vi "rocket fuel system start.vi"() -> ()   [LabVIEW 2017]
uses:
  typedefs/fuel tank.ctl
  typedefs/horiz oxidizer valve.ctl
  typedefs/oxidizer tank.ctl
  typedefs/vertical fuel valve.ctl
  typedefs/vertical oxidizer valve.ctl
  typedefs/horiz fuel valve.ctl
  typedefs/user controls.ctl
  typedefs/system state.ctl
  typedefs/sysyem status.ctl
  typedefs/rocket system warnings.ctl
panel:
  out "fuel leak w":bool
  out "fuel over w":bool
  out "system status":T1=enum."Empty & Closed"
  out "lox leak w":bool
  out "LOX over w":bool
  in  "rocket controls":T2
  out "ignition":bool
  in  "fuel leak":bool
  in  "LOX leak":bool caption="oxidizer leak"
  in  "fuel over":bool
  in  "LOX over":bool caption="oxidizer overpress"
  out "fuel dump":T3
  out "fuel return":T3
  out "fuel load":T3
  out "LOX dump":T4
  out "LOX return":T4
  out "LOX comb":T5
  out "fuel comb":T6
  out "oxidizer tank":T7 scale=0.0..100.0
  out "LOX load":T4
  out "fuel tank":T8 scale=0.0..100.0
  # "LOX\nfeed"
  # "LOX\nreturn"
  # "fuel\nfeed"
  # "fuel\nreturn"
  # "Rocket\nEngine\nFueling\nSystem\nState\nMachine"
  # "fuel\ndump"
  # "LOX\ndump"
  # "combustion\nchamber"
  # "Standard\nProcedures"
  # "Alternate\nProcedures"
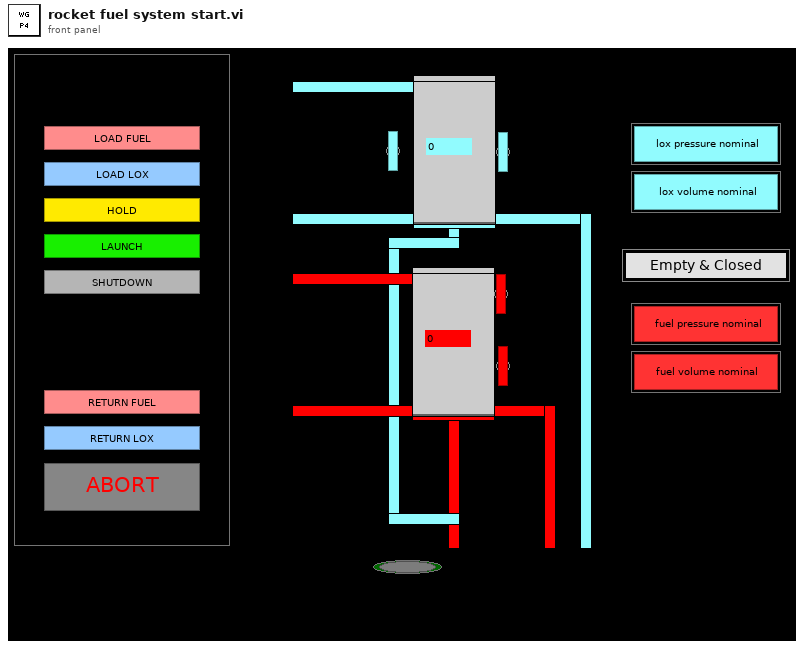
[diagram p1: front panel]
types:
  T1 = typedef "system state.ctl" = enum16{"Hold", "Empty & Closed", "Launch", "Return Fuel", "Return LOX", "Loading Lox", "Loading Fuel", "Shutdown", "Abort"}
  T2 = typedef "user controls.ctl" = cluster{"load fuel":bool, "load lox":bool, "hold":bool, "launch":bool, "shutdown":bool, "return fuel":bool, "return lox":bool, "abort":bool}
  T3 = typedef "horiz fuel valve.ctl" = u16
  T4 = typedef "horiz oxidizer valve.ctl" = u16
  T5 = typedef "vertical oxidizer valve.ctl" = u16
  T6 = typedef "vertical fuel valve.ctl" = u16
  T7 = typedef "oxidizer tank.ctl" = dbl
  T8 = typedef "fuel tank.ctl" = dbl
  T9 = typedef "sysyem status.ctl" = cluster{"system state":T1, "fuel level":dbl, "LOX level":dbl, "system warnings":T10, "valves":cluster{"fuel load":bool, "fuel return":bool, "fuel comb":bool, "fuel dump":bool, "LOX load":bool, "LOX return":bool, "LOX comb":bool, "LOX dump":bool}, "ignition":bool}
  T10 = typedef "rocket system warnings.ctl" = cluster{"oxidizer overpress":bool, "oxidizer leak":bool, "fuel overpress":bool, "fuel leak":bool}
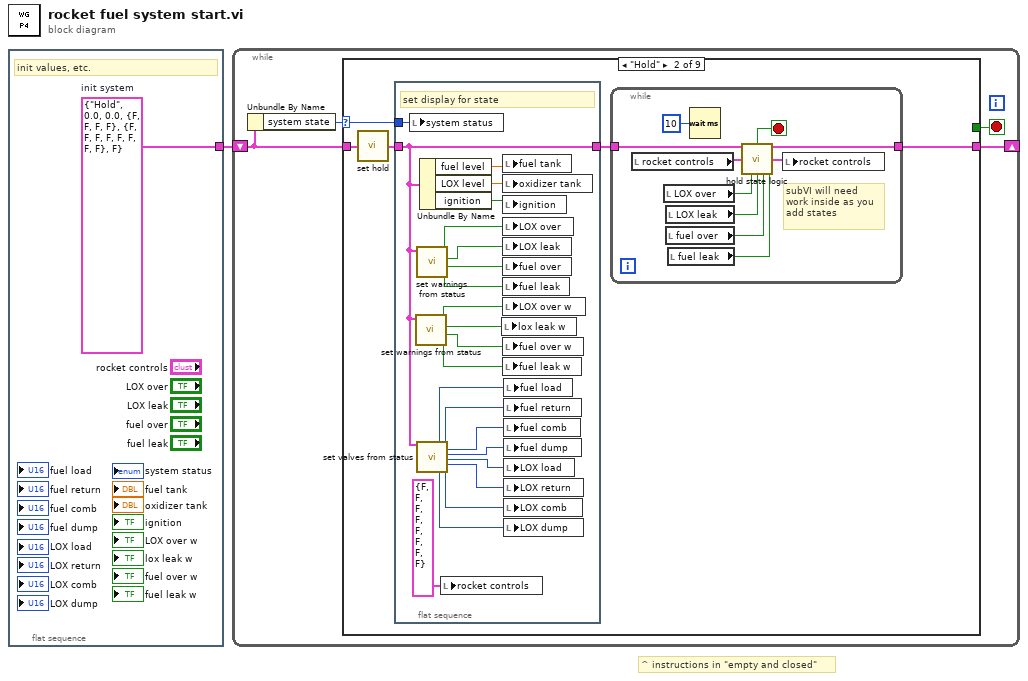
[diagram p0: block diagram]
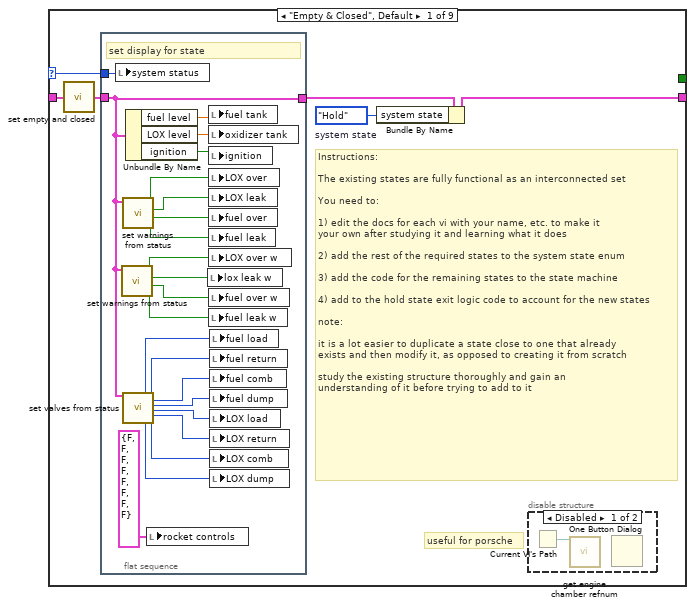
[diagram p2: hidden frame]
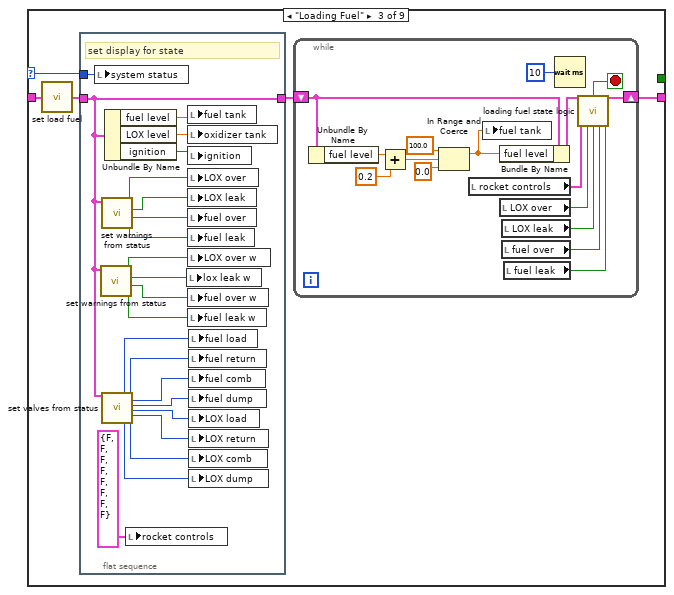
[diagram p4: hidden frame]
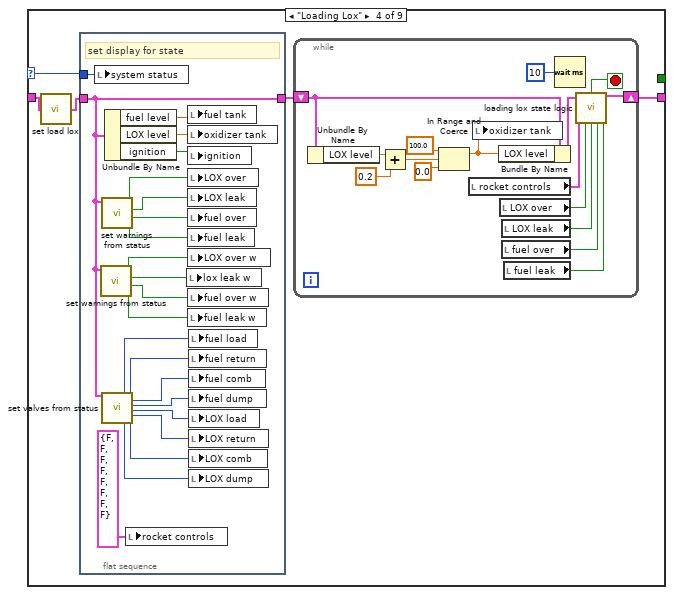
[diagram p5: hidden frame]
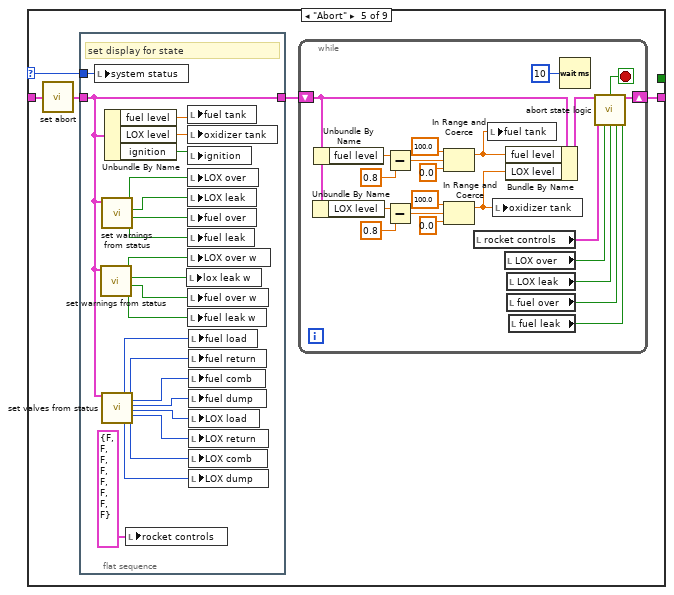
[diagram p6: hidden frame]
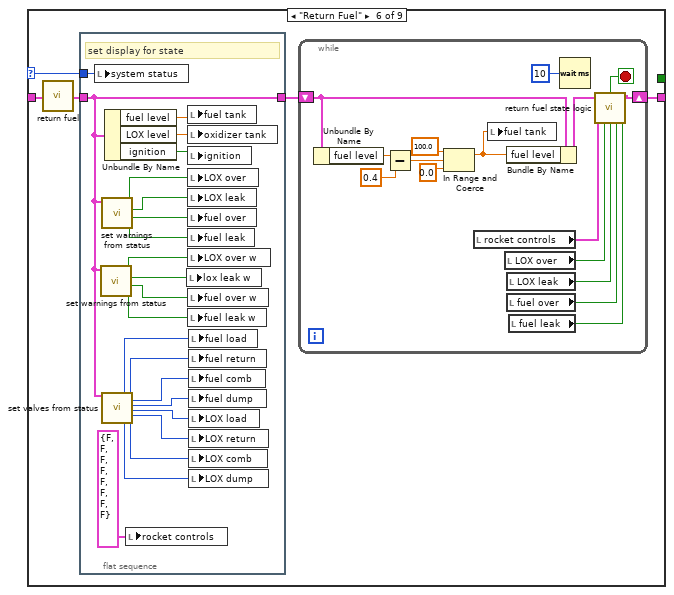
[diagram p7: hidden frame]
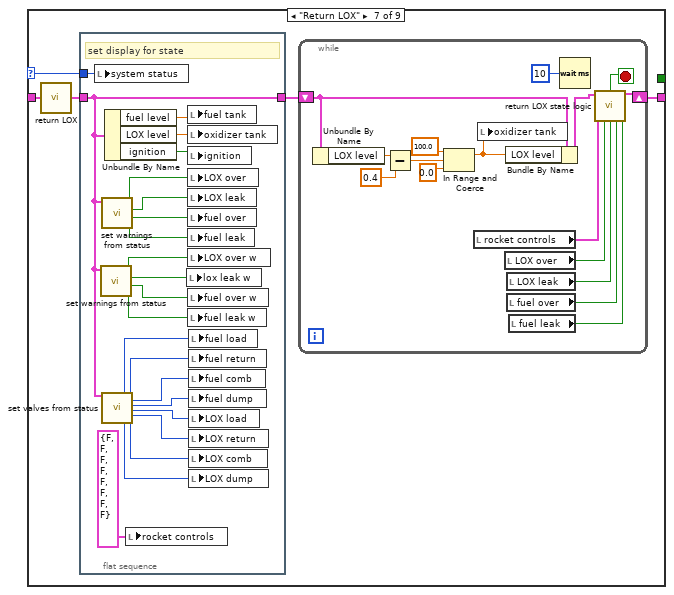
[diagram p8: hidden frame]
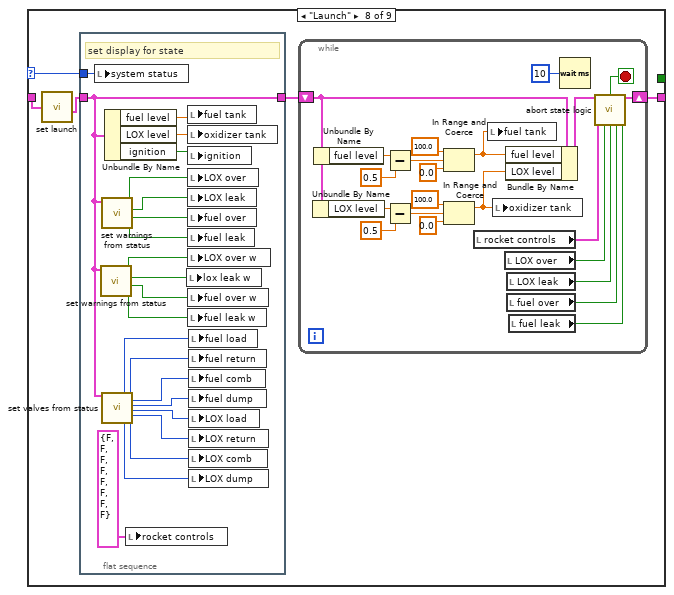
[diagram p9: hidden frame]
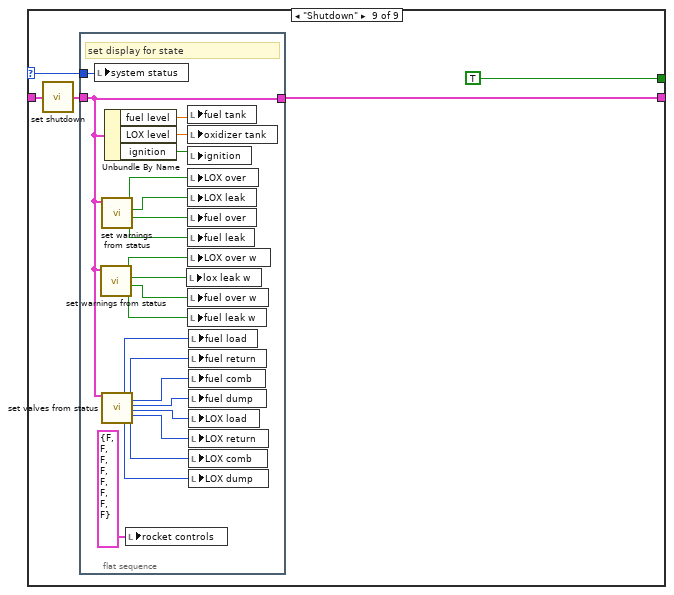
[diagram p10: hidden frame]
diagram:
  # "^ instructions in \"empty and closed\""
  n1 = flat-sequence {
    tunnel: [w2] -> w1
    frame #0 {
      w2 = T9 {"system state"=enum."Hold", "fuel level"=0.0, "LOX level"=0.0, "system warnings"={"oxidizer overpress"=FALSE, "oxidizer leak"=FALSE, "fuel overpress"=FALSE, "fuel leak"=FALSE}, "valves"={"fuel load"=FALSE, "fuel return"=FALSE, "fuel comb"=FALSE, "fuel dump"=FALSE, "LOX load"=FALSE, "LOX return"=FALSE, "LOX comb"=FALSE, "LOX dump"=FALSE}, "ignition"=FALSE}  # init system
      # "init values, etc."
    }
  }
  n2 = while {
    shift-right: [w4] -> _
    shift-left: w1 -> [w6]
    stop <- w3 stop-if-true
    n3 = Unbundle By Name(w6) -> ("system state"=w5:T1)
    n4 = case shown="\"Hold\"" w5 {
      selector: w5 -> [w12 w40 w77 w120 w163 w212 w255 w298 w347]
      tunnel: w6 -> [w10 w37 w74 w117 w162 w208 w252 w295 w346]
      tunnel: [w8 w38 w75 w118 w159 w210 w253 w296 w343] -> w4
      tunnel: [_ _ _ _ _ _ _ _ TRUE] -> w3
      frame "Empty & Closed", Default {
        w7 = system_state."Hold"  # system state
        # "useful for porsche"
        # "Instructions:\n\nThe existing states are fully functional as an interconnected set\n\nYou need to:\n\n1) edit the docs for each vi with your name, etc. to make it\nyour own after studying it and learning what it does\n\n2) add the rest of the required states to the system state enum\n\n3) add the code for the remaining states to the state machine\n\n4) add to the hold state exit logic code to account for the new states\n\nnote:\n\nit is a lot easier to duplicate a state close to one that already\nexists and then modify it, as opposed to creating it from scratch\n\nstudy the existing structure thoroughly and gain an\nunderstanding of it before trying to add to it"
        n5 = call "set empty and closed.vi"("system status in"=w10) -> ("system status out"=w9:T9)  [unwired: 14 in]
        n6 = flat-sequence {
          tunnel: w12 -> [w35]
          tunnel: w9 -> [w23]
          tunnel: [w23] -> w11
          frame #0 {
            # "set display for state"
            n7 = local write "system status"(w35) -> ()
            n8 = call "set warnings from status.vi"("system status"=w23) -> ("fuel leak w"=w24:bool, "fuel over w"=w25:bool, "lox leak w"=w27:bool, "LOX over w"=w26:bool)  [unwired: 7 in]
            n9 = call "set warnings from status.vi"("system status"=w23) -> ("fuel leak w"=w28:bool, "fuel over w"=w30:bool, "lox leak w"=w31:bool, "LOX over w"=w29:bool)  [unwired: 7 in]
            n10 = call "set valves from status.vi"("system status in"=w23) -> ("fuel load"=w22:u16, "LOX dump"=w21:u16, "fuel return"=w20:u16, "fuel comb"=w16:u16, "fuel dump"=w18:u16, "LOX load"=w17:u16, "LOX return"=w15:u16, "LOX comb"=w19:u16)  [unwired: 11 in]
            n11 = Unbundle By Name(w23) -> ("fuel level"=w33:dbl, "LOX level"=w34:dbl, "ignition"=w32:bool)
            n12 = local write "rocket controls"(T2 {"load fuel"=FALSE, "load lox"=FALSE, "hold"=FALSE, "launch"=FALSE, "shutdown"=FALSE, "return fuel"=FALSE, "return lox"=FALSE, "abort"=FALSE} ("rocket controls")) -> ()
            n13 = local write "lox leak w"(w27) -> ()
            n14 = local write "fuel tank"(w33) -> ()
            n15 = local write "oxidizer tank"(w34) -> ()
            n16 = local write "ignition"(w32) -> ()
            n17 = local write "LOX over"(w29) -> ()
            n18 = local write "LOX leak"(w31) -> ()
            n19 = local write "fuel over"(w30) -> ()
            n20 = local write "fuel leak"(w28) -> ()
            n21 = local write "LOX over w"(w26) -> ()
            n22 = local write "fuel over w"(w25) -> ()
            n23 = local write "fuel leak w"(w24) -> ()
            n24 = local write "fuel load"(w22) -> ()
            n25 = local write "fuel return"(w20) -> ()
            n26 = local write "fuel comb"(w16) -> ()
            n27 = local write "fuel dump"(w18) -> ()
            n28 = local write "LOX load"(w17) -> ()
            n29 = local write "LOX return"(w15) -> ()
            n30 = local write "LOX comb"(w19) -> ()
            n31 = local write "LOX dump"(w21) -> ()
          }
        }
        n32 = Bundle By Name(cluster=w11, "system state"=w7) -> (w8:T9)
        n33 = disable-structure shown="Disabled" {
          frame Disabled {
            n34 = Current VI's Path() -> (path=w13:path)
            n35 = call "get engine chamber refnum.vi"("this vi path"=w13) -> ()  [unwired: 14 in, 1 out]
            n36 = One Button Dialog() -> ()  [unwired: 2 in, 1 out]
          }
          frame Enabled {
          }
        }
      }
      frame "Hold" {
        n37 = call "set hold.vi"("system status in"=w37) -> ("system status out"=w36:T9)  [unwired: 14 in]
        n38 = flat-sequence {
          tunnel: w40 -> [w72]
          tunnel: [w51] -> w39
          tunnel: w36 -> [w51]
          frame #0 {
            # "set display for state"
            n39 = local write "system status"(w72) -> ()
            n40 = call "set warnings from status.vi"("system status"=w51) -> ("fuel leak w"=w61:bool, "fuel over w"=w62:bool, "lox leak w"=w64:bool, "LOX over w"=w63:bool)  [unwired: 7 in]
            n41 = call "set warnings from status.vi"("system status"=w51) -> ("fuel leak w"=w65:bool, "fuel over w"=w67:bool, "lox leak w"=w68:bool, "LOX over w"=w66:bool)  [unwired: 7 in]
            n42 = call "set valves from status.vi"("system status in"=w51) -> ("fuel load"=w60:u16, "LOX dump"=w59:u16, "fuel return"=w58:u16, "fuel comb"=w54:u16, "fuel dump"=w56:u16, "LOX load"=w55:u16, "LOX return"=w53:u16, "LOX comb"=w57:u16)  [unwired: 11 in]
            n43 = Unbundle By Name(w51) -> ("fuel level"=w70:dbl, "LOX level"=w71:dbl, "ignition"=w69:bool)
            n44 = local write "rocket controls"(T2 {"load fuel"=FALSE, "load lox"=FALSE, "hold"=FALSE, "launch"=FALSE, "shutdown"=FALSE, "return fuel"=FALSE, "return lox"=FALSE, "abort"=FALSE} ("rocket controls")) -> ()
            n45 = local write "lox leak w"(w64) -> ()
            n46 = local write "fuel tank"(w70) -> ()
            n47 = local write "oxidizer tank"(w71) -> ()
            n48 = local write "ignition"(w69) -> ()
            n49 = local write "LOX over"(w66) -> ()
            n50 = local write "LOX leak"(w68) -> ()
            n51 = local write "fuel over"(w67) -> ()
            n52 = local write "fuel leak"(w65) -> ()
            n53 = local write "LOX over w"(w63) -> ()
            n54 = local write "fuel over w"(w62) -> ()
            n55 = local write "fuel leak w"(w61) -> ()
            n56 = local write "fuel load"(w60) -> ()
            n57 = local write "fuel return"(w58) -> ()
            n58 = local write "fuel comb"(w54) -> ()
            n59 = local write "fuel dump"(w56) -> ()
            n60 = local write "LOX load"(w55) -> ()
            n61 = local write "LOX return"(w53) -> ()
            n62 = local write "LOX comb"(w57) -> ()
            n63 = local write "LOX dump"(w59) -> ()
          }
        }
        n64 = while {
          tunnel: w39 -> [w49]
          tunnel: [w48] -> w38
          stop <- w43 stop-if-true
          # "subVI will need \nwork inside as you\nadd states"
          n65 = local read "rocket controls"() -> (w41:T2)
          n66 = local read "LOX over"() -> (w44:bool)
          n67 = local read "LOX leak"() -> (w45:bool)
          n68 = local read "fuel over"() -> (w46:bool)
          n69 = local read "fuel leak"() -> (w47:bool)
          n70 = Wait (ms)(milliseconds to wait=u32 10) -> ()  [unwired: 1 out]
          n71 = call "hold state logic.vi"("system status in"=w49, "rocket controls"=w41, "LOX over"=w44, "LOX leak"=w45, "fuel over"=w46, "fuel leak"=w47) -> ("stop hold loop"=w43:bool, "system status out"=w48:T9, "rocket controls out"=w42:T2)  [unwired: 7 in]
          n72 = local write "rocket controls"(w42) -> ()
        }
      }
      frame "Loading Fuel" {
        n73 = call "set load fuel.vi"("system status in"=w74) -> ("system status out"=w73:T9)  [unwired: 14 in]
        n74 = flat-sequence {
          tunnel: w77 -> [w115]
          tunnel: [w94] -> w76
          tunnel: w73 -> [w94]
          frame #0 {
            # "set display for state"
            n75 = local write "system status"(w115) -> ()
            n76 = call "set warnings from status.vi"("system status"=w94) -> ("fuel leak w"=w104:bool, "fuel over w"=w105:bool, "lox leak w"=w107:bool, "LOX over w"=w106:bool)  [unwired: 7 in]
            n77 = call "set warnings from status.vi"("system status"=w94) -> ("fuel leak w"=w108:bool, "fuel over w"=w110:bool, "lox leak w"=w111:bool, "LOX over w"=w109:bool)  [unwired: 7 in]
            n78 = call "set valves from status.vi"("system status in"=w94) -> ("fuel load"=w103:u16, "LOX dump"=w102:u16, "fuel return"=w101:u16, "fuel comb"=w97:u16, "fuel dump"=w99:u16, "LOX load"=w98:u16, "LOX return"=w96:u16, "LOX comb"=w100:u16)  [unwired: 11 in]
            n79 = Unbundle By Name(w94) -> ("fuel level"=w113:dbl, "LOX level"=w114:dbl, "ignition"=w112:bool)
            n80 = local write "rocket controls"(T2 {"load fuel"=FALSE, "load lox"=FALSE, "hold"=FALSE, "launch"=FALSE, "shutdown"=FALSE, "return fuel"=FALSE, "return lox"=FALSE, "abort"=FALSE} ("rocket controls")) -> ()
            n81 = local write "lox leak w"(w107) -> ()
            n82 = local write "fuel tank"(w113) -> ()
            n83 = local write "oxidizer tank"(w114) -> ()
            n84 = local write "ignition"(w112) -> ()
            n85 = local write "LOX over"(w109) -> ()
            n86 = local write "LOX leak"(w111) -> ()
            n87 = local write "fuel over"(w110) -> ()
            n88 = local write "fuel leak"(w108) -> ()
            n89 = local write "LOX over w"(w106) -> ()
            n90 = local write "fuel over w"(w105) -> ()
            n91 = local write "fuel leak w"(w104) -> ()
            n92 = local write "fuel load"(w103) -> ()
            n93 = local write "fuel return"(w101) -> ()
            n94 = local write "fuel comb"(w97) -> ()
            n95 = local write "fuel dump"(w99) -> ()
            n96 = local write "LOX load"(w98) -> ()
            n97 = local write "LOX return"(w96) -> ()
            n98 = local write "LOX comb"(w100) -> ()
            n99 = local write "LOX dump"(w102) -> ()
          }
        }
        n100 = while {
          shift-right: [w92] -> w75
          shift-left: w76 -> [w85]
          stop <- w91 stop-if-true
          n101 = Unbundle By Name(w85) -> ("fuel level"=w83:dbl)
          n102 = Add(x=w83, y=0.2) -> (x+y=w81:dbl)
          n103 = In Range and Coerce(upper limit=100.0, x=w81, lower limit=0.0) -> (coerced(x)=w78:dbl)  [unwired: 1 out]
          n104 = local read "rocket controls"() -> (w90:T2)
          n105 = local write "fuel tank"(w78) -> ()
          n106 = Bundle By Name(cluster=w85, "fuel level"=w78) -> (w84:T9)
          n107 = local read "LOX over"() -> (w89:bool)
          n108 = local read "LOX leak"() -> (w88:bool)
          n109 = local read "fuel over"() -> (w87:bool)
          n110 = local read "fuel leak"() -> (w86:bool)
          n111 = Wait (ms)(milliseconds to wait=u32 10) -> ()  [unwired: 1 out]
          n112 = call "loading fuel state logic.vi"("system status in"=w84, "rocket controls"=w90, "LOX over"=w89, "LOX leak"=w88, "fuel over"=w87, "fuel leak"=w86) -> ("stop loop"=w91:bool, "system status out"=w92:T9)  [unwired: 8 in]
        }
      }
      frame "Loading Lox" {
        n113 = call "set load lox.vi"("system status in"=w117) -> ("system status out"=w116:T9)  [unwired: 14 in]
        n114 = flat-sequence {
          tunnel: w120 -> [w158]
          tunnel: [w137] -> w119
          tunnel: w116 -> [w137]
          frame #0 {
            # "set display for state"
            n115 = local write "system status"(w158) -> ()
            n116 = call "set warnings from status.vi"("system status"=w137) -> ("fuel leak w"=w147:bool, "fuel over w"=w148:bool, "lox leak w"=w150:bool, "LOX over w"=w149:bool)  [unwired: 7 in]
            n117 = call "set warnings from status.vi"("system status"=w137) -> ("fuel leak w"=w151:bool, "fuel over w"=w153:bool, "lox leak w"=w154:bool, "LOX over w"=w152:bool)  [unwired: 7 in]
            n118 = call "set valves from status.vi"("system status in"=w137) -> ("fuel load"=w146:u16, "LOX dump"=w145:u16, "fuel return"=w144:u16, "fuel comb"=w140:u16, "fuel dump"=w142:u16, "LOX load"=w141:u16, "LOX return"=w139:u16, "LOX comb"=w143:u16)  [unwired: 11 in]
            n119 = Unbundle By Name(w137) -> ("fuel level"=w156:dbl, "LOX level"=w157:dbl, "ignition"=w155:bool)
            n120 = local write "rocket controls"(T2 {"load fuel"=FALSE, "load lox"=FALSE, "hold"=FALSE, "launch"=FALSE, "shutdown"=FALSE, "return fuel"=FALSE, "return lox"=FALSE, "abort"=FALSE} ("rocket controls")) -> ()
            n121 = local write "lox leak w"(w150) -> ()
            n122 = local write "fuel tank"(w156) -> ()
            n123 = local write "oxidizer tank"(w157) -> ()
            n124 = local write "ignition"(w155) -> ()
            n125 = local write "LOX over"(w152) -> ()
            n126 = local write "LOX leak"(w154) -> ()
            n127 = local write "fuel over"(w153) -> ()
            n128 = local write "fuel leak"(w151) -> ()
            n129 = local write "LOX over w"(w149) -> ()
            n130 = local write "fuel over w"(w148) -> ()
            n131 = local write "fuel leak w"(w147) -> ()
            n132 = local write "fuel load"(w146) -> ()
            n133 = local write "fuel return"(w144) -> ()
            n134 = local write "fuel comb"(w140) -> ()
            n135 = local write "fuel dump"(w142) -> ()
            n136 = local write "LOX load"(w141) -> ()
            n137 = local write "LOX return"(w139) -> ()
            n138 = local write "LOX comb"(w143) -> ()
            n139 = local write "LOX dump"(w145) -> ()
          }
        }
        n140 = while {
          shift-right: [w122] -> w118
          shift-left: w119 -> [w135]
          stop <- w121 stop-if-true
          n141 = Unbundle By Name(w135) -> ("LOX level"=w134:dbl)
          n142 = Add(x=w134, y=0.2) -> (x+y=w132:dbl)
          n143 = In Range and Coerce(upper limit=100.0, x=w132, lower limit=0.0) -> (coerced(x)=w129:dbl)  [unwired: 1 out]
          n144 = local read "rocket controls"() -> (w127:T2)
          n145 = local write "oxidizer tank"(w129) -> ()
          n146 = Bundle By Name(cluster=w135, "LOX level"=w129) -> (w128:T9)
          n147 = local read "LOX over"() -> (w123:bool)
          n148 = local read "LOX leak"() -> (w124:bool)
          n149 = local read "fuel over"() -> (w125:bool)
          n150 = local read "fuel leak"() -> (w126:bool)
          n151 = Wait (ms)(milliseconds to wait=u32 10) -> ()  [unwired: 1 out]
          n152 = call "loading lox state logic.vi"("system status in"=w128, "rocket controls"=w127, "LOX over"=w123, "LOX leak"=w124, "fuel over"=w125, "fuel leak"=w126) -> ("stop loop"=w121:bool, "system status out"=w122:T9)  [unwired: 8 in]
        }
      }
      frame "Abort" {
        n153 = call "set abort.vi"("system status in"=w162) -> ("system status out"=w161:T9)  [unwired: 14 in]
        n154 = flat-sequence {
          tunnel: w163 -> [w207]
          tunnel: [w186] -> w160
          tunnel: w161 -> [w186]
          frame #0 {
            # "set display for state"
            n155 = local write "system status"(w207) -> ()
            n156 = call "set warnings from status.vi"("system status"=w186) -> ("fuel leak w"=w196:bool, "fuel over w"=w197:bool, "lox leak w"=w199:bool, "LOX over w"=w198:bool)  [unwired: 7 in]
            n157 = call "set warnings from status.vi"("system status"=w186) -> ("fuel leak w"=w200:bool, "fuel over w"=w202:bool, "lox leak w"=w203:bool, "LOX over w"=w201:bool)  [unwired: 7 in]
            n158 = call "set valves from status.vi"("system status in"=w186) -> ("fuel load"=w195:u16, "LOX dump"=w194:u16, "fuel return"=w193:u16, "fuel comb"=w189:u16, "fuel dump"=w191:u16, "LOX load"=w190:u16, "LOX return"=w188:u16, "LOX comb"=w192:u16)  [unwired: 11 in]
            n159 = Unbundle By Name(w186) -> ("fuel level"=w205:dbl, "LOX level"=w206:dbl, "ignition"=w204:bool)
            n160 = local write "rocket controls"(T2 {"load fuel"=FALSE, "load lox"=FALSE, "hold"=FALSE, "launch"=FALSE, "shutdown"=FALSE, "return fuel"=FALSE, "return lox"=FALSE, "abort"=FALSE} ("rocket controls")) -> ()
            n161 = local write "lox leak w"(w199) -> ()
            n162 = local write "fuel tank"(w205) -> ()
            n163 = local write "oxidizer tank"(w206) -> ()
            n164 = local write "ignition"(w204) -> ()
            n165 = local write "LOX over"(w201) -> ()
            n166 = local write "LOX leak"(w203) -> ()
            n167 = local write "fuel over"(w202) -> ()
            n168 = local write "fuel leak"(w200) -> ()
            n169 = local write "LOX over w"(w198) -> ()
            n170 = local write "fuel over w"(w197) -> ()
            n171 = local write "fuel leak w"(w196) -> ()
            n172 = local write "fuel load"(w195) -> ()
            n173 = local write "fuel return"(w193) -> ()
            n174 = local write "fuel comb"(w189) -> ()
            n175 = local write "fuel dump"(w191) -> ()
            n176 = local write "LOX load"(w190) -> ()
            n177 = local write "LOX return"(w188) -> ()
            n178 = local write "LOX comb"(w192) -> ()
            n179 = local write "LOX dump"(w194) -> ()
          }
        }
        n180 = while {
          shift-right: [w184] -> w159
          shift-left: w160 -> [w164]
          stop <- w183 stop-if-true
          n181 = Unbundle By Name(w164) -> ("LOX level"=w166:dbl)
          n182 = Unbundle By Name(w164) -> ("fuel level"=w176:dbl)
          n183 = Subtract(x=w176, y=0.8) -> (x-y=w174:dbl)
          n184 = Subtract(x=w166, y=0.8) -> (x-y=w168:dbl)
          n185 = In Range and Coerce(upper limit=100.0, x=w174, lower limit=0.0) -> (coerced(x)=w171:dbl)  [unwired: 1 out]
          n186 = In Range and Coerce(upper limit=100.0, x=w168, lower limit=0.0) -> (coerced(x)=w165:dbl)  [unwired: 1 out]
          n187 = local read "rocket controls"() -> (w182:T2)
          n188 = local write "fuel tank"(w171) -> ()
          n189 = local write "oxidizer tank"(w165) -> ()
          n190 = local read "LOX over"() -> (w181:bool)
          n191 = Bundle By Name(cluster=w164, "fuel level"=w171, "LOX level"=w165) -> (w177:T9)
          n192 = local read "LOX leak"() -> (w180:bool)
          n193 = local read "fuel over"() -> (w179:bool)
          n194 = local read "fuel leak"() -> (w178:bool)
          n195 = Wait (ms)(milliseconds to wait=u32 10) -> ()  [unwired: 1 out]
          n196 = call "abort state logic.vi"("system status in"=w177, "rocket controls"=w182, "LOX over"=w181, "LOX leak"=w180, "fuel over"=w179, "fuel leak"=w178) -> ("stop loop"=w183:bool, "system status out"=w184:T9)  [unwired: 8 in]
        }
      }
      frame "Return Fuel" {
        n197 = call "return fuel.vi"("system status in"=w208) -> ("system status out"=w209:T9)  [unwired: 14 in]
        n198 = flat-sequence {
          tunnel: w212 -> [w250]
          tunnel: [w229] -> w211
          tunnel: w209 -> [w229]
          frame #0 {
            # "set display for state"
            n199 = local write "system status"(w250) -> ()
            n200 = call "set warnings from status.vi"("system status"=w229) -> ("fuel leak w"=w239:bool, "fuel over w"=w240:bool, "lox leak w"=w242:bool, "LOX over w"=w241:bool)  [unwired: 7 in]
            n201 = call "set warnings from status.vi"("system status"=w229) -> ("fuel leak w"=w243:bool, "fuel over w"=w245:bool, "lox leak w"=w246:bool, "LOX over w"=w244:bool)  [unwired: 7 in]
            n202 = call "set valves from status.vi"("system status in"=w229) -> ("fuel load"=w238:u16, "LOX dump"=w237:u16, "fuel return"=w236:u16, "fuel comb"=w232:u16, "fuel dump"=w234:u16, "LOX load"=w233:u16, "LOX return"=w231:u16, "LOX comb"=w235:u16)  [unwired: 11 in]
            n203 = Unbundle By Name(w229) -> ("fuel level"=w248:dbl, "LOX level"=w249:dbl, "ignition"=w247:bool)
            n204 = local write "rocket controls"(T2 {"load fuel"=FALSE, "load lox"=FALSE, "hold"=FALSE, "launch"=FALSE, "shutdown"=FALSE, "return fuel"=FALSE, "return lox"=FALSE, "abort"=FALSE} ("rocket controls")) -> ()
            n205 = local write "lox leak w"(w242) -> ()
            n206 = local write "fuel tank"(w248) -> ()
            n207 = local write "oxidizer tank"(w249) -> ()
            n208 = local write "ignition"(w247) -> ()
            n209 = local write "LOX over"(w244) -> ()
            n210 = local write "LOX leak"(w246) -> ()
            n211 = local write "fuel over"(w245) -> ()
            n212 = local write "fuel leak"(w243) -> ()
            n213 = local write "LOX over w"(w241) -> ()
            n214 = local write "fuel over w"(w240) -> ()
            n215 = local write "fuel leak w"(w239) -> ()
            n216 = local write "fuel load"(w238) -> ()
            n217 = local write "fuel return"(w236) -> ()
            n218 = local write "fuel comb"(w232) -> ()
            n219 = local write "fuel dump"(w234) -> ()
            n220 = local write "LOX load"(w233) -> ()
            n221 = local write "LOX return"(w231) -> ()
            n222 = local write "LOX comb"(w235) -> ()
            n223 = local write "LOX dump"(w237) -> ()
          }
        }
        n224 = while {
          shift-right: [w213] -> w210
          shift-left: w211 -> [w221]
          stop <- w214 stop-if-true
          n225 = Unbundle By Name(w221) -> ("fuel level"=w227:dbl)
          n226 = Subtract(x=w227, y=0.4) -> (x-y=w225:dbl)
          n227 = In Range and Coerce(upper limit=100.0, x=w225, lower limit=0.0) -> (coerced(x)=w222:dbl)  [unwired: 1 out]
          n228 = local read "rocket controls"() -> (w219:T2)
          n229 = local write "fuel tank"(w222) -> ()
          n230 = local read "LOX over"() -> (w218:bool)
          n231 = Bundle By Name(cluster=w221, "fuel level"=w222) -> (w220:T9)
          n232 = local read "LOX leak"() -> (w217:bool)
          n233 = local read "fuel over"() -> (w216:bool)
          n234 = local read "fuel leak"() -> (w215:bool)
          n235 = Wait (ms)(milliseconds to wait=u32 10) -> ()  [unwired: 1 out]
          n236 = call "return fuel state logic.vi"("system status in"=w220, "rocket controls"=w219, "LOX over"=w218, "LOX leak"=w217, "fuel over"=w216, "fuel leak"=w215) -> ("stop loop"=w214:bool, "system status out"=w213:T9)  [unwired: 8 in]
        }
      }
      frame "Return LOX" {
        n237 = call "return LOX.vi"("system status in"=w252) -> ("system status out"=w251:T9)  [unwired: 14 in]
        n238 = flat-sequence {
          tunnel: w255 -> [w293]
          tunnel: [w272] -> w254
          tunnel: w251 -> [w272]
          frame #0 {
            # "set display for state"
            n239 = local write "system status"(w293) -> ()
            n240 = call "set warnings from status.vi"("system status"=w272) -> ("fuel leak w"=w282:bool, "fuel over w"=w283:bool, "lox leak w"=w285:bool, "LOX over w"=w284:bool)  [unwired: 7 in]
            n241 = call "set warnings from status.vi"("system status"=w272) -> ("fuel leak w"=w286:bool, "fuel over w"=w288:bool, "lox leak w"=w289:bool, "LOX over w"=w287:bool)  [unwired: 7 in]
            n242 = call "set valves from status.vi"("system status in"=w272) -> ("fuel load"=w281:u16, "LOX dump"=w280:u16, "fuel return"=w279:u16, "fuel comb"=w275:u16, "fuel dump"=w277:u16, "LOX load"=w276:u16, "LOX return"=w274:u16, "LOX comb"=w278:u16)  [unwired: 11 in]
            n243 = Unbundle By Name(w272) -> ("fuel level"=w291:dbl, "LOX level"=w292:dbl, "ignition"=w290:bool)
            n244 = local write "rocket controls"(T2 {"load fuel"=FALSE, "load lox"=FALSE, "hold"=FALSE, "launch"=FALSE, "shutdown"=FALSE, "return fuel"=FALSE, "return lox"=FALSE, "abort"=FALSE} ("rocket controls")) -> ()
            n245 = local write "lox leak w"(w285) -> ()
            n246 = local write "fuel tank"(w291) -> ()
            n247 = local write "oxidizer tank"(w292) -> ()
            n248 = local write "ignition"(w290) -> ()
            n249 = local write "LOX over"(w287) -> ()
            n250 = local write "LOX leak"(w289) -> ()
            n251 = local write "fuel over"(w288) -> ()
            n252 = local write "fuel leak"(w286) -> ()
            n253 = local write "LOX over w"(w284) -> ()
            n254 = local write "fuel over w"(w283) -> ()
            n255 = local write "fuel leak w"(w282) -> ()
            n256 = local write "fuel load"(w281) -> ()
            n257 = local write "fuel return"(w279) -> ()
            n258 = local write "fuel comb"(w275) -> ()
            n259 = local write "fuel dump"(w277) -> ()
            n260 = local write "LOX load"(w276) -> ()
            n261 = local write "LOX return"(w274) -> ()
            n262 = local write "LOX comb"(w278) -> ()
            n263 = local write "LOX dump"(w280) -> ()
          }
        }
        n264 = while {
          shift-right: [w256] -> w253
          shift-left: w254 -> [w264]
          stop <- w257 stop-if-true
          n265 = Unbundle By Name(w264) -> ("LOX level"=w270:dbl)
          n266 = Subtract(x=w270, y=0.4) -> (x-y=w268:dbl)
          n267 = In Range and Coerce(upper limit=100.0, x=w268, lower limit=0.0) -> (coerced(x)=w265:dbl)  [unwired: 1 out]
          n268 = local read "rocket controls"() -> (w262:T2)
          n269 = local write "oxidizer tank"(w265) -> ()
          n270 = local read "LOX over"() -> (w261:bool)
          n271 = Bundle By Name(cluster=w264, "LOX level"=w265) -> (w263:T9)
          n272 = local read "LOX leak"() -> (w260:bool)
          n273 = local read "fuel over"() -> (w259:bool)
          n274 = local read "fuel leak"() -> (w258:bool)
          n275 = Wait (ms)(milliseconds to wait=u32 10) -> ()  [unwired: 1 out]
          n276 = call "return LOX state logic.vi"("system status in"=w263, "rocket controls"=w262, "LOX over"=w261, "LOX leak"=w260, "fuel over"=w259, "fuel leak"=w258) -> ("stop loop"=w257:bool, "system status out"=w256:T9)  [unwired: 8 in]
        }
      }
      frame "Launch" {
        n277 = call "set launch.vi"("system status in"=w295) -> ("system status out"=w294:T9)  [unwired: 14 in]
        n278 = flat-sequence {
          tunnel: w298 -> [w342]
          tunnel: [w321] -> w297
          tunnel: w294 -> [w321]
          frame #0 {
            # "set display for state"
            n279 = local write "system status"(w342) -> ()
            n280 = call "set warnings from status.vi"("system status"=w321) -> ("fuel leak w"=w331:bool, "fuel over w"=w332:bool, "lox leak w"=w334:bool, "LOX over w"=w333:bool)  [unwired: 7 in]
            n281 = call "set warnings from status.vi"("system status"=w321) -> ("fuel leak w"=w335:bool, "fuel over w"=w337:bool, "lox leak w"=w338:bool, "LOX over w"=w336:bool)  [unwired: 7 in]
            n282 = call "set valves from status.vi"("system status in"=w321) -> ("fuel load"=w330:u16, "LOX dump"=w329:u16, "fuel return"=w328:u16, "fuel comb"=w324:u16, "fuel dump"=w326:u16, "LOX load"=w325:u16, "LOX return"=w323:u16, "LOX comb"=w327:u16)  [unwired: 11 in]
            n283 = Unbundle By Name(w321) -> ("fuel level"=w340:dbl, "LOX level"=w341:dbl, "ignition"=w339:bool)
            n284 = local write "rocket controls"(T2 {"load fuel"=FALSE, "load lox"=FALSE, "hold"=FALSE, "launch"=FALSE, "shutdown"=FALSE, "return fuel"=FALSE, "return lox"=FALSE, "abort"=FALSE} ("rocket controls")) -> ()
            n285 = local write "lox leak w"(w334) -> ()
            n286 = local write "fuel tank"(w340) -> ()
            n287 = local write "oxidizer tank"(w341) -> ()
            n288 = local write "ignition"(w339) -> ()
            n289 = local write "LOX over"(w336) -> ()
            n290 = local write "LOX leak"(w338) -> ()
            n291 = local write "fuel over"(w337) -> ()
            n292 = local write "fuel leak"(w335) -> ()
            n293 = local write "LOX over w"(w333) -> ()
            n294 = local write "fuel over w"(w332) -> ()
            n295 = local write "fuel leak w"(w331) -> ()
            n296 = local write "fuel load"(w330) -> ()
            n297 = local write "fuel return"(w328) -> ()
            n298 = local write "fuel comb"(w324) -> ()
            n299 = local write "fuel dump"(w326) -> ()
            n300 = local write "LOX load"(w325) -> ()
            n301 = local write "LOX return"(w323) -> ()
            n302 = local write "LOX comb"(w327) -> ()
            n303 = local write "LOX dump"(w329) -> ()
          }
        }
        n304 = while {
          shift-right: [w319] -> w296
          shift-left: w297 -> [w299]
          stop <- w318 stop-if-true
          n305 = Unbundle By Name(w299) -> ("LOX level"=w301:dbl)
          n306 = Unbundle By Name(w299) -> ("fuel level"=w311:dbl)
          n307 = Subtract(x=w311, y=0.5) -> (x-y=w309:dbl)
          n308 = Subtract(x=w301, y=0.5) -> (x-y=w303:dbl)
          n309 = In Range and Coerce(upper limit=100.0, x=w309, lower limit=0.0) -> (coerced(x)=w306:dbl)  [unwired: 1 out]
          n310 = In Range and Coerce(upper limit=100.0, x=w303, lower limit=0.0) -> (coerced(x)=w300:dbl)  [unwired: 1 out]
          n311 = local read "rocket controls"() -> (w317:T2)
          n312 = local write "fuel tank"(w306) -> ()
          n313 = local write "oxidizer tank"(w300) -> ()
          n314 = local read "LOX over"() -> (w316:bool)
          n315 = Bundle By Name(cluster=w299, "fuel level"=w306, "LOX level"=w300) -> (w312:T9)
          n316 = local read "LOX leak"() -> (w315:bool)
          n317 = local read "fuel over"() -> (w314:bool)
          n318 = local read "fuel leak"() -> (w313:bool)
          n319 = Wait (ms)(milliseconds to wait=u32 10) -> ()  [unwired: 1 out]
          n320 = call "abort state logic.vi"("system status in"=w312, "rocket controls"=w317, "LOX over"=w316, "LOX leak"=w315, "fuel over"=w314, "fuel leak"=w313) -> ("stop loop"=w318:bool, "system status out"=w319:T9)  [unwired: 8 in]
        }
      }
      frame "Shutdown" {
        n321 = call "set shutdown.vi"("system status in"=w346) -> ("system status out"=w345:T9)  [unwired: 14 in]
        n322 = flat-sequence {
          tunnel: w347 -> [w369]
          tunnel: w345 -> [w357]
          tunnel: [w357] -> w343
          frame #0 {
            # "set display for state"
            n323 = local write "system status"(w369) -> ()
            n324 = call "set warnings from status.vi"("system status"=w357) -> ("fuel leak w"=w358:bool, "fuel over w"=w359:bool, "lox leak w"=w361:bool, "LOX over w"=w360:bool)  [unwired: 7 in]
            n325 = call "set warnings from status.vi"("system status"=w357) -> ("fuel leak w"=w362:bool, "fuel over w"=w364:bool, "lox leak w"=w365:bool, "LOX over w"=w363:bool)  [unwired: 7 in]
            n326 = call "set valves from status.vi"("system status in"=w357) -> ("fuel load"=w356:u16, "LOX dump"=w355:u16, "fuel return"=w354:u16, "fuel comb"=w350:u16, "fuel dump"=w352:u16, "LOX load"=w351:u16, "LOX return"=w349:u16, "LOX comb"=w353:u16)  [unwired: 11 in]
            n327 = Unbundle By Name(w357) -> ("fuel level"=w367:dbl, "LOX level"=w368:dbl, "ignition"=w366:bool)
            n328 = local write "rocket controls"(T2 {"load fuel"=FALSE, "load lox"=FALSE, "hold"=FALSE, "launch"=FALSE, "shutdown"=FALSE, "return fuel"=FALSE, "return lox"=FALSE, "abort"=FALSE} ("rocket controls")) -> ()
            n329 = local write "lox leak w"(w361) -> ()
            n330 = local write "fuel tank"(w367) -> ()
            n331 = local write "oxidizer tank"(w368) -> ()
            n332 = local write "ignition"(w366) -> ()
            n333 = local write "LOX over"(w363) -> ()
            n334 = local write "LOX leak"(w365) -> ()
            n335 = local write "fuel over"(w364) -> ()
            n336 = local write "fuel leak"(w362) -> ()
            n337 = local write "LOX over w"(w360) -> ()
            n338 = local write "fuel over w"(w359) -> ()
            n339 = local write "fuel leak w"(w358) -> ()
            n340 = local write "fuel load"(w356) -> ()
            n341 = local write "fuel return"(w354) -> ()
            n342 = local write "fuel comb"(w350) -> ()
            n343 = local write "fuel dump"(w352) -> ()
            n344 = local write "LOX load"(w351) -> ()
            n345 = local write "LOX return"(w349) -> ()
            n346 = local write "LOX comb"(w353) -> ()
            n347 = local write "LOX dump"(w355) -> ()
          }
        }
      }
    }
  }
